vi "Assert Cal Attendance.vi"() -> ()   [LabVIEW 2015, in "Admin_Actor.lvlib" / "CalAttendance.lvclass"]
uses:
  CalAttendance.lvclass
  Type Definitions/NumOfAttendace.ctl
  API/_Database/Database.lvclass
  CalAttendance.lvclass/CalAttendance.ctl
panel:
  out "NumOfAttendance":T1
  out "Res_Attendance":cluster{"BackGround":u32, "Reason":string}[][](array[cluster])
  out "Names(\"\") 2":string[](array[string])
  out "Names(\"\")":string[](array[string])
  out "Departments(\"\")":string[](array[string])
  in  "path":path=path "E:/哈工大竞技机器人队/机器人队管理系统/Database/CRTDatabase.accdb"
  in  "ExcusePath":path=path "E:/哈工大竞技机器人队/机器人队管理系统/Database/考勤报表.xls"
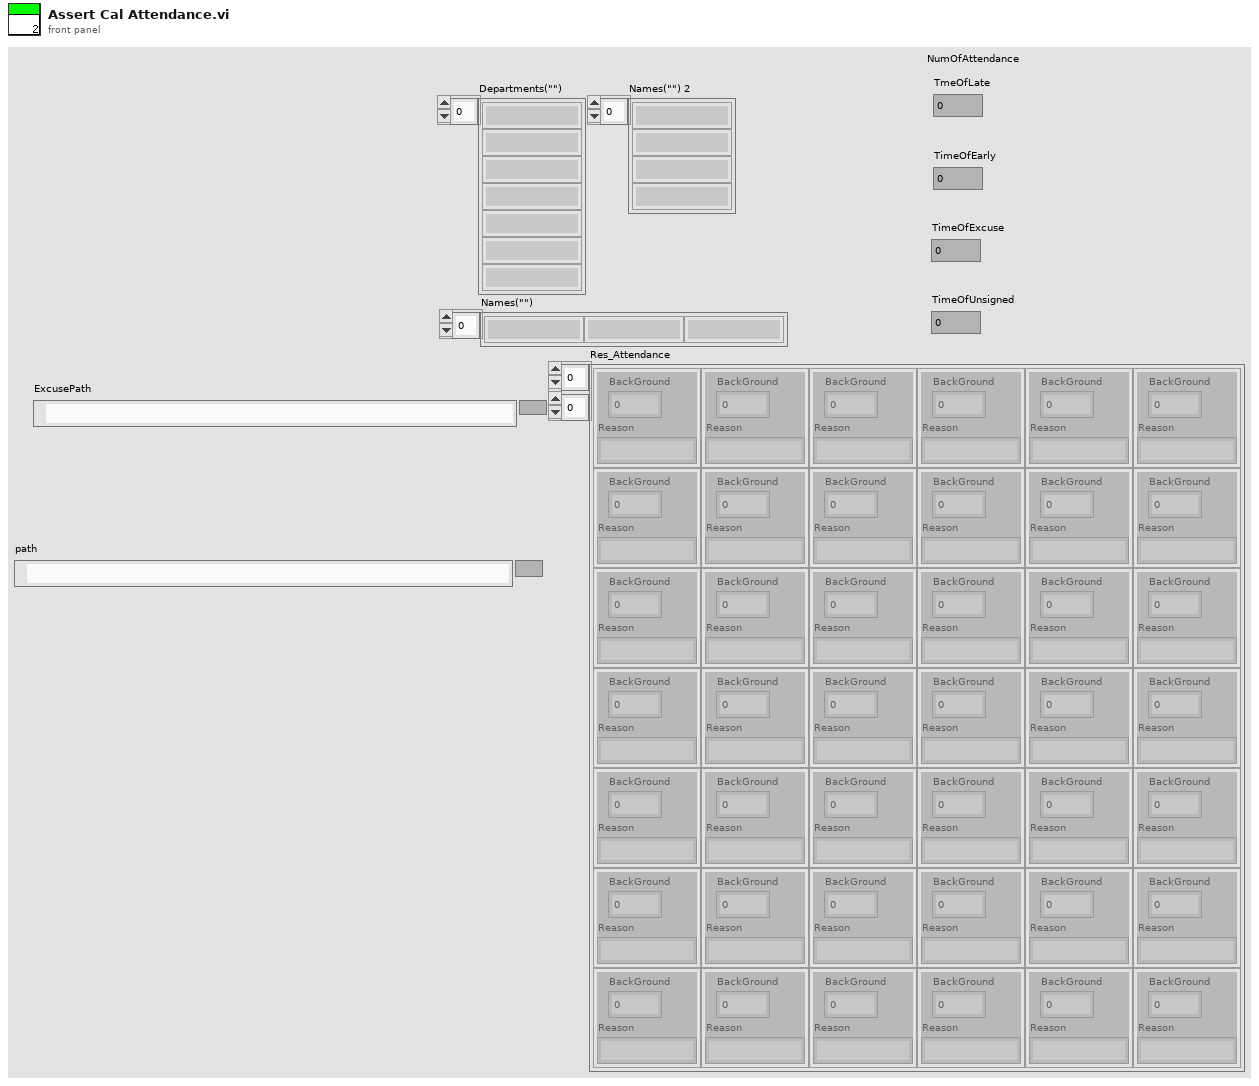
[diagram p1: front panel]
types:
  T1 = typedef "Admin_Actor.lvlib/CalAttendance.lvclass/NumOfAttendace.ctl" = cluster{"TmeOfLate":i32, "TimeOfEarly":i32, "TimeOfExcuse":i32, "TimeOfUnsigned":i32}
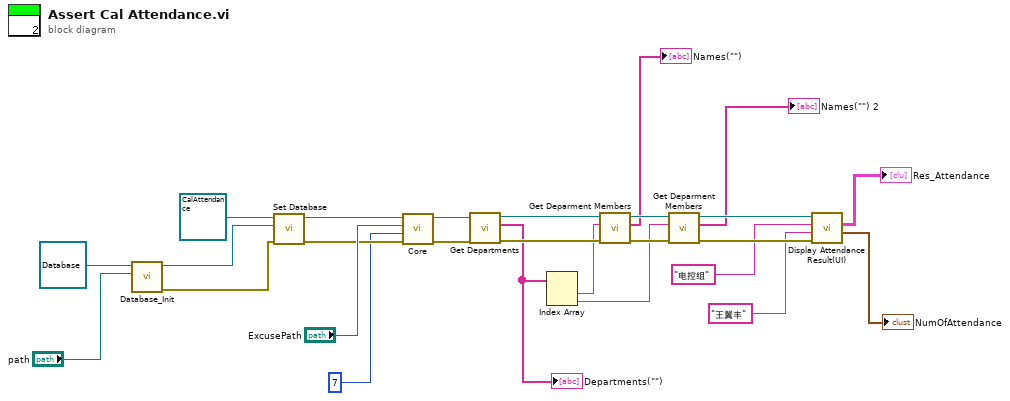
[diagram p0: block diagram]
diagram:
  n1 = call "Database_Init.vi"("path"="path", "object in"=refnum<class "Database.lvclass"> refnum ("Database")) -> ("error out"=w21:errorcluster, "object out"=w22:refnum<class "Database.lvclass">)  [unwired: 8 in]
  n2 = call "Set Database.vi"("error in (no error)"=w21, "Database"=w22, "CalAttendance in"=refnum<class "CalAttendance.lvclass"> refnum) -> ("error out"=w19:errorcluster, "CalAttendance out"=w20:refnum<class "CalAttendance.lvclass">)  [unwired: 7 in]
  n3 = call "Core.vi"("error in (no error)"=w19, "CurWeek(0)"=7, "ExcusePath"="ExcusePath", "CalAttendance in"=w20) -> ("error out"=w16:errorcluster, "CalAttendance out"=w17:refnum<class "CalAttendance.lvclass">)  [unwired: 6 in]
  n4 = call "Get Departments.vi"("error in (no error)"=w16, "CalAttendance in"=w17) -> ("error out"=w14:errorcluster, "Departments(\"\")"=w13:string[], "CalAttendance out"=w15:refnum<class "CalAttendance.lvclass">)  [unwired: 7 in]
  "Departments(\"\")" <- w13
  n5 = Index Array(array=w13) -> (element #1=w7:string, element #2=w6:string)  [unwired: 2 in]
  n6 = call "Get Deparment Members.vi"("error in (no error)"=w14, "Department(\"\")"=w7, "CalAttendance in"=w15) -> ("error out"=w11:errorcluster, "Names(\"\")"=→"Names(\"\")":string[], "CalAttendance out"=w12:refnum<class "CalAttendance.lvclass">)  [unwired: 6 in]
  n7 = call "Get Deparment Members.vi"("error in (no error)"=w11, "Department(\"\")"=w6, "CalAttendance in"=w12) -> ("error out"=w8:errorcluster, "Names(\"\")"=→"Names(\"\") 2":string[], "CalAttendance out"=w9:refnum<class "CalAttendance.lvclass">)  [unwired: 6 in]
  n8 = call "Display Attendance Result(UI).vi"("error in (no error)"=w8, "Name(\"\")"="王翼丰" ("Name(\"\")"), "Department(\"\")"="电控组" ("Department(\"\")"), "CalAttendance in"=w9) -> ("NumOfAttendance"=→"NumOfAttendance":T1, "Res_Attendance"=→"Res_Attendance":cluster{"BackGround":u32, "Reason":string}[][])  [unwired: 4 in, 2 out]
